vi "Del Graph.vi"(5 "file name":string) -> (1 "read string":string, 2 "Del successful?":bool)   [LabVIEW 2009]
uses:
  Global/Global 1.vi
panel:
  out "existing?":bool
  out "match substring":string
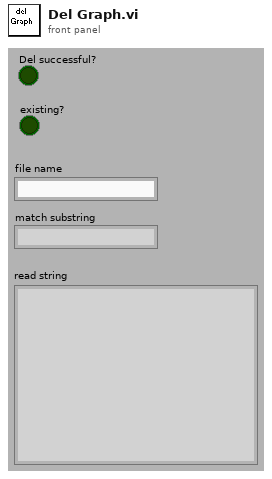
[diagram p1: front panel]
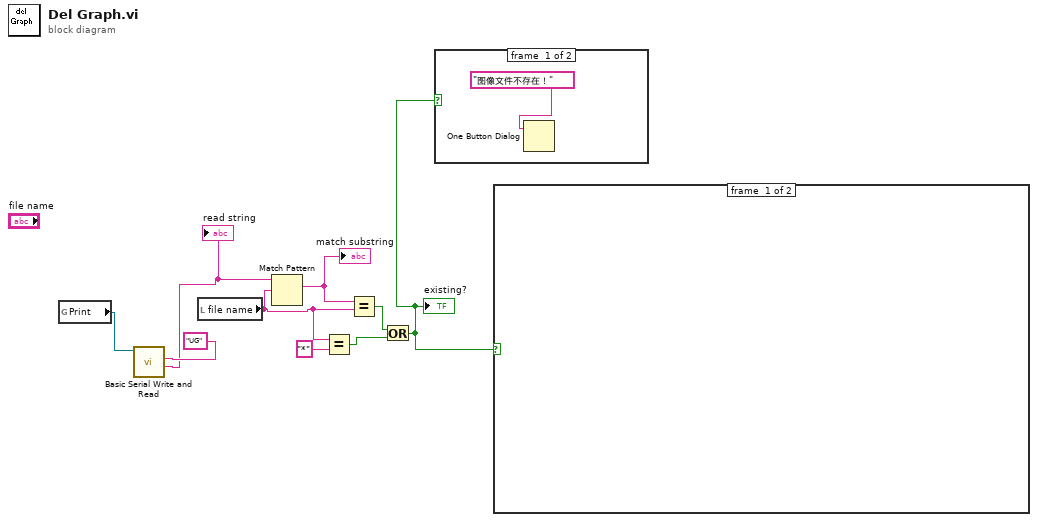
[diagram p0: block diagram]
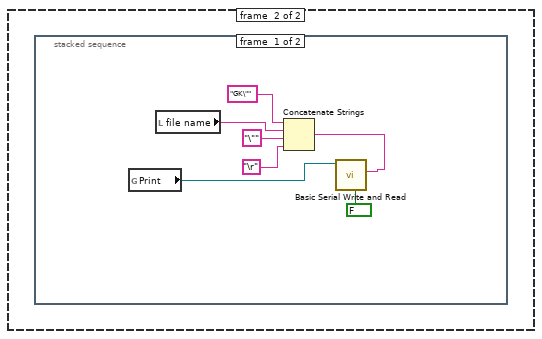
[diagram p3: hidden frame]
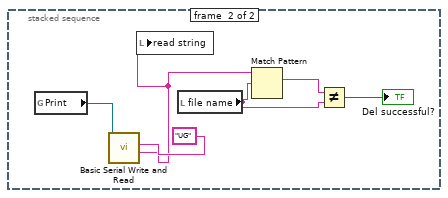
[diagram p4: hidden frame]
diagram:
  n1 = global read "Global 1.vi" "Print"() -> (w1:refnum<visa-resource-name>)
  n2 = call "Basic Serial Write and Read.vi"("VISA resource name"=w1, "string to write"="UG") -> ("read string"=w2:string)  [unwired: 7 in, 1 out]
  "read string" <- w2
  n3 = local read "file name"() -> (w8:string)
  n4 = Match Pattern(string=w2, regular expression=w8) -> (match substring=w9:string)  [unwired: 4 out]
  "match substring" <- w9
  n5 = Equal?(x=w8, y="*") -> (x = y?=w5:bool)
  n6 = Equal?(x=w9, y=w8) -> (x = y?=w6:bool)
  n7 = Or(x=w6, y=w5) -> (x .or. y?=w4:bool)
  "existing?" <- w4
  n8 = case shown="True" w4 {
    frame #0 {
      n9 = One Button Dialog(message="图像文件不存在！") -> ()  [unwired: 2 out]
    }
    frame #1 {
    }
  }
  n10 = case shown="True" w4 {
    frame #0 {
    }
    frame #1 {
      n11 = stacked-sequence {
        frame #0 {
          n12 = global read "Global 1.vi" "Print"() -> (w11:refnum<visa-resource-name>)
          n13 = local read "file name"() -> (w15:string)
          n14 = Concatenate Strings("GK\"" ("string"), w15, "\"" ("string"), "\r") -> (w13:string)
          n15 = call "Basic Serial Write and Read.vi"("VISA resource name"=w11, "read"=FALSE, "string to write"=w13) -> ()  [unwired: 6 in, 2 out]
        }
        frame #1 {
          n16 = global read "Global 1.vi" "Print"() -> (w18:refnum<visa-resource-name>)
          n17 = call "Basic Serial Write and Read.vi"("VISA resource name"=w18, "string to write"="UG") -> ("read string"=w19:string)  [unwired: 7 in, 1 out]
          n18 = local write "read string"(w19) -> ()
          n19 = local read "file name"() -> (w23:string)
          n20 = Match Pattern(string=w19, regular expression=w23) -> (match substring=w22:string)  [unwired: 4 out]
          n21 = Not Equal?(x=w22, y=w23) -> (x != y?=→"Del successful?":bool)
        }
      }
    }
  }
